vi "buffer calling.vi"() -> ()   [LabVIEW 2019]
panel:
  out "buffer out":dbl[](array[numeric]) format="%.2f"
  in  "Iteration":u16
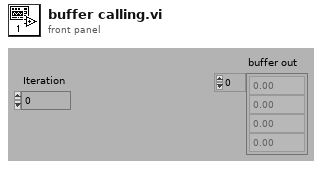
[diagram p1: front panel]
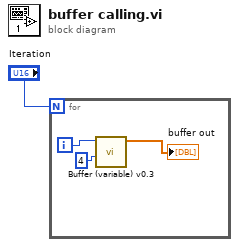
[diagram p0: block diagram]
diagram:
  n1 = for {
    N: "Iteration" -> [_]
    i -> [w4]
    n2 = call "Buffer (variable) v0.3.vi"("Max Buffer Size"=4, "Numeric"=w4) -> ("Buffer"=→"buffer out":dbl[])  [unwired: 9 in]
  }
